vi "New.vi"(6 "Delimiters":T1={"Close"="}}", "Open"="{{"}, 8 "Error In":errorcluster, 11 "Content":string) -> (0 "Error Out":errorcluster, 3 "Comment":refnum<class "Comment.lvclass">)   [LabVIEW 2018, in "Toolkit.lvlib" / "Tokens.lvlib" / "Comment.lvclass"]
doc: "Creates a new Comment object."
uses:
  Comment.lvclass
  Type Definitions/Delimiters.ctl
  Toolkit.lvlib
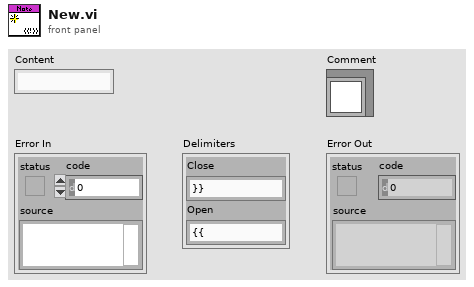
[diagram p1: front panel]
types:
  T1 = typedef "Toolkit.lvlib/Delimiters.ctl" = cluster{"Close":string, "Open":string}
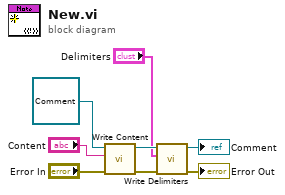
[diagram p0: block diagram]
diagram:
  n1 = call-dynamic "Write Content.vi"("Error In"="Error In", "Content"="Content", "Contentable In"=refnum<class "Comment.lvclass"> refnum ("Toolkit.lvlib:Tokens.lvlib:Comment.lvclass")) -> ("Error Out"=w2:errorcluster, "Contentable Out"=w5:refnum<class "Comment.lvclass">)  [unwired: 7 in]
  n2 = call-dynamic "Write Delimiters.vi"("Error In"=w2, "Delimiters"="Delimiters", "Token In"=w5) -> ("Error Out"=→"Error Out":errorcluster, "Token Out"=→"Comment":refnum<class "Comment.lvclass">)  [unwired: 7 in]
